vi "Forward Kinematics.vi"() -> ()   [LabVIEW 2018]
uses:
  <vilib>/Platform/TimedLoop/XDataNode/timing_clust.ctl
  <vilib>/Platform/TimedLoop/XDataNode/nitl_modes.ctl
  <vilib>/Platform/TimedLoop/XDataNode/wakeup.ctl
  <extravilib>/ChannelInstances/Tag-bool/Read With Abort.vi
  <extravilib>/ChannelInstances/Tag-bool/Write With Abort.vi
  <extravilib>/ChannelInstances/Tag-bool/Instantiate.vi
  <extravilib>/ChannelInstances/Tag-bool/EndpointRead.vi
  <extravilib>/ChannelInstances/Tag-bool/Endpoint.vi
  <vilib>/Platform/TimedLoop/XDataNode/XDataNode.xnode
  <vilib>/Platform/TimedLoop/XDataNode/XDNodeRunTimeDep.lvlib
  <extravilib>/ChannelInstances/Tag-bool.lvlib
panel:
  out "Camera Image":T1(plugin-control)
  in  "Stop Button":bool
  out "Calibrated":bool
  out "End-effector Trajectory":cluster{dbl[], dbl[]}[](graph)
  out "Task Coordinates (cm)":dbl[](array[numeric])
  out "Joint Coordinates (rad)":dbl[](array[numeric])
  out "E theta (rad)":dbl
  # "Engineering Trainer Boards"
  # "Forward Kinematics"
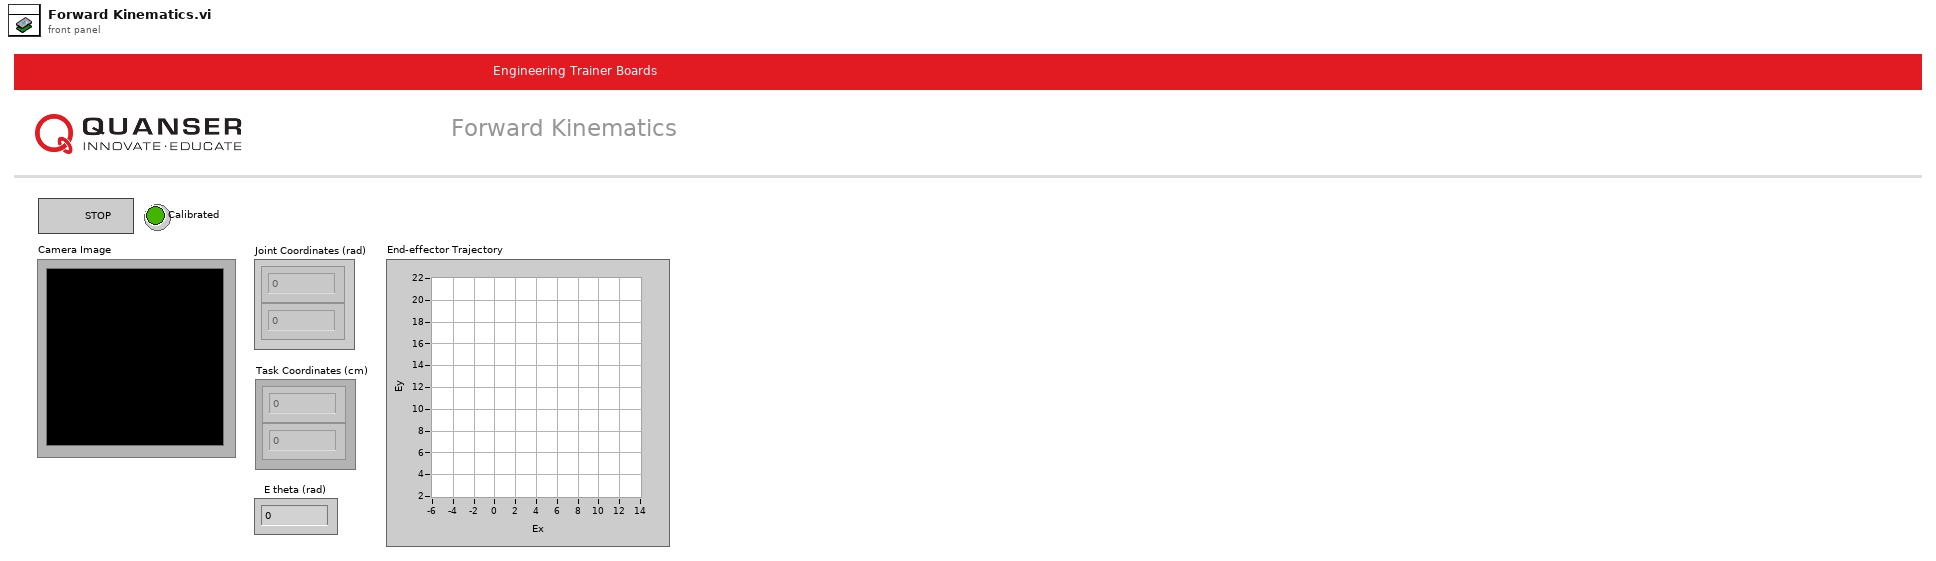
[diagram p1: front panel]
types:
  T1 = typedef "IMAQ Image.ctl" = refnum<image>
  T2 = typedef "XDNodeRunTimeDep.lvlib/timing_clust.ctl" = cluster{"Expected End [f-1]":u64, "Actual End [f-1]":u64, "Finished Late? [f-1]":bool, "Expected End [i-1]":u64, "Actual End [i-1]":u64, "Finished Late? [i-1]":bool, "Expected Start [i]":u64, "Actual Start [i]":u64, "Expected Start [f]":u64, "Actual Start [f]":u64, "Source Name":string, "Structure Name":string, "Period":i64, "Deadline":i64, "Offset":i64, "Start":i64, "Priority":i32, "Timeout":i32, "Mode":T3, "Wakeup Reason":T4, "Error":errorcluster, "Source Type":string, "Secondary Source Type":string, "Global End Time":u64, "Global Start Time":u64, "Frame Duration":u64, "Iteration Duration":u64, "Assigned CPU":i32, "I/O Scan Engine Mode":u32}
  T3 = typedef "XDNodeRunTimeDep.lvlib/nitl_modes.ctl" = enum32{"No Change", "Process missed periods, maintain original phase", "Discard missed periods, maintain original phase", "Process missed periods, ignore original phase", "Discard missed periods, ignore original phase"}
  T4 = typedef "XDNodeRunTimeDep.lvlib/wakeup.ctl" = enum32{"Normal", "Aborted", "Asynchronous wakeup", "Timing source error", "Timed loop error", "Timeout"}
  T5 = typedef "QNET MS IO Cluster.ctl" = cluster{"Error":errorcluster, "Encoder Calibration Values":i32[], "Update Calibration":bool, "JPEG Resolutions":u16, "Raw Resolutions":u16, "Image Mode":enum16{"RAW RGB", "RAW Gray Scale", "JPEG"}, "FPGA Ref":refnum<k20>}
  T6 = typedef "Tag-bool.lvlib/))Channel.ctl" = refnum<queue>
  T7 = cluster{"Left":i32, "Top":i32, "Right":i32, "Bottom":i32}
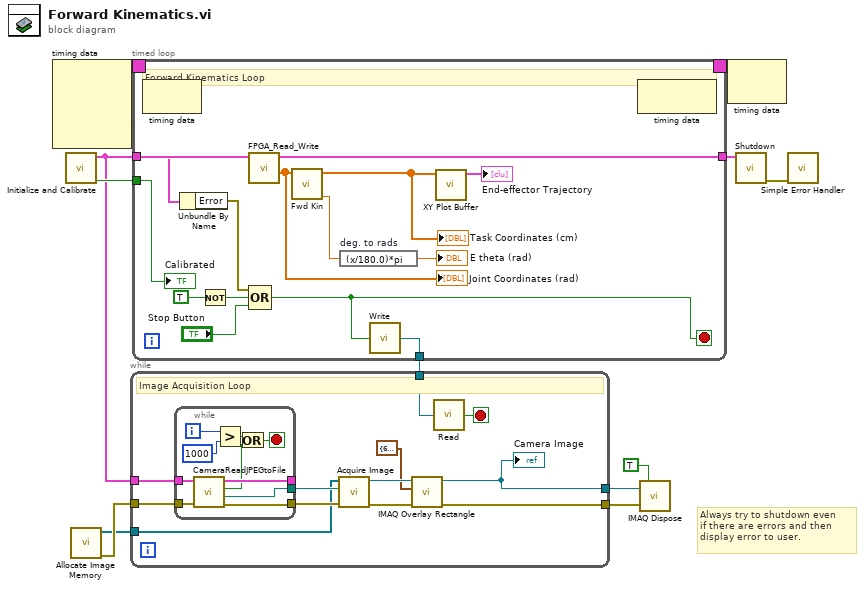
[diagram p0: block diagram]
diagram:
  # "Always try to shutdown even \nif there are errors and then \ndisplay error to user."
  n1 = node-c288() -> (w12:T2)  [unwired: 4 in]
  n2 = call "Initialize and Calibrate.vi"() -> ("Calibrated"=w8:bool, "IO Cluster"=w2:T5)  [unwired: 10 in]
  n3 = call "Allocate Image Memory.vi"() -> ("error out"=w7:errorcluster, "Acquisition Memory"=w6:T1[])  [unwired: 6 in, 4 out]
  n4 = timed-loop {
    timing: w12 -> [_]
    timing-out: [_] -> w11
    tunnel: w2 -> [w23]
    tunnel: [w20] -> w9
    tunnel: w8 -> [w19]
    tunnel: [w14] -> w1
    stop <- w17 stop-if-true
    # "Forward Kinematics Loop"
    n5 = node-c288() -> ()  [unwired: 1 in, 1 out]
    n6 = Not(x=TRUE) -> (.not. x?=w18:bool)
    n7 = call "FPGA_Read_Write.vi"("IO Cluster In"=w23) -> ("Joint Coordinates (rad)"=w26:dbl[], "IO Cluster Out"=w20:T5)  [unwired: 7 in, 2 out]
    "Joint Coordinates (rad)" <- w26
    n8 = Unbundle By Name(w20) -> ("Error"=w15:errorcluster)
    n9 = Compound Arithmetic op=OR(w15, w18, "Stop Button") -> (w17:bool)
    n10 = call "Fwd Kin.vi"("Joint Coordinates (rad)"=w26) -> ("E_theta (deg)"=w25:dbl, "Task Coordinates (cm)"=w21:dbl[])  [unwired: 9 in]
    "Task Coordinates (cm)" <- w21
    n11 = expression code="(x/180.0)*pi" "deg. to rads"(w25) -> (→"E theta (rad)":dbl)
    n12 = call <extravilib>:"Write.vi"("element"=w17) -> ("channel"=w14:T6)  [unwired: 1 out]
    n13 = call "XY Plot Buffer.vi"("Actual"=w21) -> ("Buffered Task Coordinates"=→"End-effector Trajectory":cluster{dbl[], dbl[]}[])  [unwired: 10 in]
    n14 = node-c288() -> ()  [unwired: 1 in, 1 out]
    "Calibrated" <- w19
  }
  n15 = while {
    tunnel: w2 -> [w38]
    tunnel: w7 -> [w37]
    tunnel: w6 -> [w36]
    tunnel: [w32] -> w3
    tunnel: [w30] -> w4
    tunnel: w1 -> [w35]
    stop <- w34 stop-if-true
    # "Image Acquisition Loop"
    n16 = while {
      tunnel: [w46] -> w39
      tunnel: w38 -> [w50]
      tunnel: [w49] -> _
      tunnel: w37 -> [w47]
      tunnel: [w48] -> w40
      i -> [w42]
      stop <- w45 stop-if-true
      n17 = call "CameraReadJPEGtoFile.vi"("error in"=w47, "IO Cluster In"=w50) -> ("Error Out"=w48:errorcluster, "Image File"=w46:path, "New Image Data"=w41:bool, "IO Cluster Out"=w49:T5)  [unwired: 6 in]
      n18 = Greater?(x=w42, y=1000) -> (0:w44:bool)
      n19 = Or(x=w44, y=w41) -> (x .or. y?=w45:bool)
    }
    n20 = call "Acquire Image.vi"("Error In"=w40, "File Path"=w39, "Acquisition Memory"=w36) -> ("Error Out"=w33:errorcluster, "Pre-processed Image"=w31:T1)  [unwired: 4 in, 3 out]
    n21 = call "IMAQ Overlay Rectangle"("error in (no error)"=w33, "Rectangle"=T7 {"Left"=60, "Top"=60, "Right"=68, "Bottom"=68}, "Image"=w31) -> ("error out"=w32:errorcluster, "Image Out"=w30:T1)  [unwired: 7 in]
    "Camera Image" <- w30
    n22 = call <extravilib>:"Read.vi"("channel"=w35) -> ("element"=w34:bool)  [unwired: 1 in, 1 out]
  }
  n23 = call "IMAQ Dispose"("All Images? (No)"=TRUE, "Image"=w4, "error in (no error)"=w3) -> ()  [unwired: 3 in, 1 out]
  n24 = node-c288(w11) -> ()  [unwired: 1 out]
  n25 = call "Shutdown.vi"("IO Cluster In"=w9) -> ("Error"=w10:errorcluster)  [unwired: 10 in]
  n26 = call <vilib>:"Simple Error Handler.vi"("error in (no error)"=w10) -> ()  [unwired: 4 in, 5 out]
